vi "lj_obtain_resources.vi"(8 "error in (no error)":errorcluster) -> (0 "error out":errorcluster, 3 "LabJackRes":T1)   [LabVIEW 2025, in "LabJackEKG.lvlib"]
uses:
  LabJackEKG.lvlib
  Typedefs/LabJackGlobalResources.ctl
  Typedefs/CounterQueues.ctl
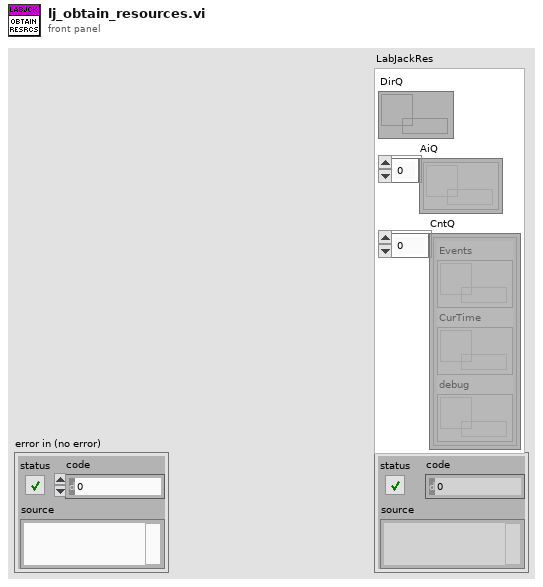
[diagram p1: front panel]
types:
  T1 = typedef "LabJackEKG.lvlib/LabJackGlobalResources.ctl" = cluster{"DirQ":refnum<queue>, "AiQ":refnum<queue>[], "CntQ":T2[]}
  T2 = typedef "LabJackEKG.lvlib/CounterQueues.ctl" = cluster{"Events":refnum<queue>, "CurTime":refnum<queue>, "debug":refnum<queue>}
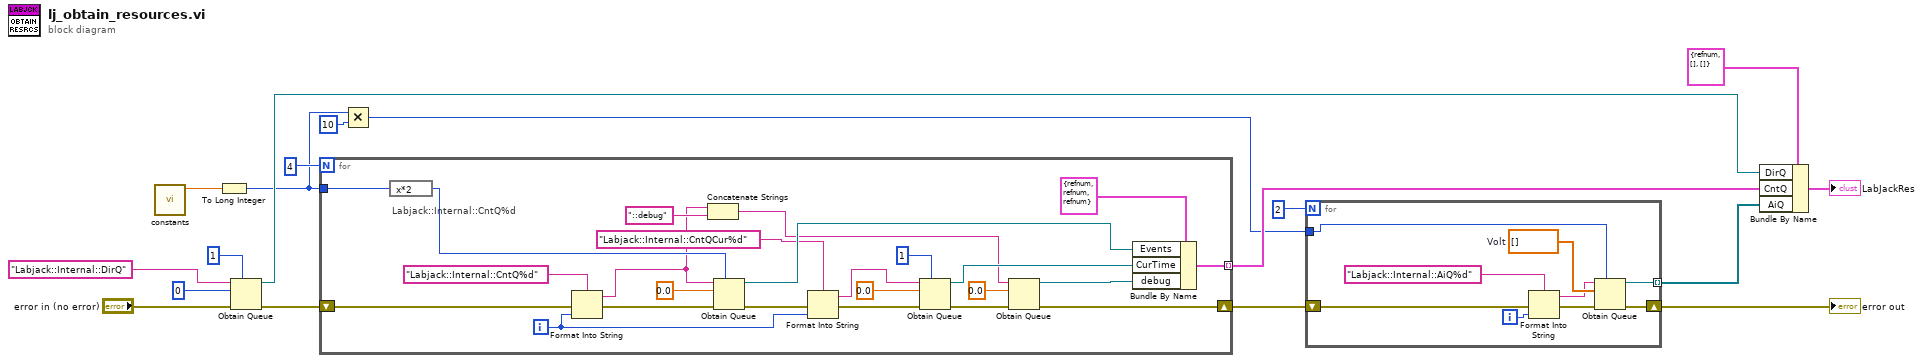
[diagram p0: block diagram]
diagram:
  n1 = call "constants.vi"() -> ("Sampling Frequency [Hz]"=w2:dbl)  [unwired: 10 in, 1 out]
  n2 = To Long Integer(number=w2) -> (32bit integer=w4:i32)
  n3 = Obtain Queue(max queue size (-1, unlimited)=1, name (unnamed)="Labjack::Internal::DirQ", element data type=i64 0, error in (no error)="error in (no error)") -> (queue out=w5:refnum<queue>, error out=w14:errorcluster)  [unwired: 1 in, 1 out]
  n4 = for {
    N: 4 -> [_]
    tunnel: [w35] -> w9 mode=indexing
    shift-right: [w29] -> w13
    shift-left: w14 -> [w40]
    tunnel: w4 -> [w33]
    i -> [w19]
    # "Labjack::Internal::CntQ%d"
    n5 = expression code="x*2"(w33) -> (w32:i32)
    n6 = Format Into String(format string="Labjack::Internal::CntQ%d", error in=w40, w19) -> (resulting string=w23:string, error out=w39:errorcluster)  [unwired: 1 in]
    n7 = Concatenate Strings(w23, "::debug" ("string")) -> (w24:string)
    n8 = Obtain Queue(max queue size (-1, unlimited)=w32, name (unnamed)=w23, element data type=0.0, error in (no error)=w39) -> (queue out=w34:refnum<queue>, error out=w42:errorcluster)  [unwired: 1 in, 1 out]
    n9 = Format Into String(format string="Labjack::Internal::CntQCur%d", error in=w42, w19) -> (resulting string=w20:string, error out=w22:errorcluster)  [unwired: 1 in]
    n10 = Obtain Queue(max queue size (-1, unlimited)=1, name (unnamed)=w20, element data type=0.0, error in (no error)=w22) -> (queue out=w31:refnum<queue>, error out=w30:errorcluster)  [unwired: 1 in, 1 out]
    n11 = Obtain Queue(name (unnamed)=w24, element data type=0.0, error in (no error)=w30) -> (queue out=w28:refnum<queue>, error out=w29:errorcluster)  [unwired: 2 in, 1 out]
    n12 = Bundle By Name(cluster=T2 {"Events"=refnum, "CurTime"=refnum, "debug"=refnum} ("CntQ 2"), "Events"=w34, "CurTime"=w31, "debug"=w28) -> (w35:T2)
  }
  n13 = Multiply(x=w4, y=10 ("max queue size (-1, unlimited)")) -> (x*y=w3:i32)
  n14 = for {
    N: 2 -> [_]
    tunnel: [w50] -> w8 mode=indexing
    shift-right: [w49] -> w12
    shift-left: w13 -> [w48]
    tunnel: w3 -> [w43]
    i -> [w46]
    w51 = dbl[] []  # Volt
    n15 = Format Into String(format string="Labjack::Internal::AiQ%d", error in=w48, w46) -> (resulting string=w44:string, error out=w47:errorcluster)  [unwired: 1 in]
    n16 = Obtain Queue(max queue size (-1, unlimited)=w43, name (unnamed)=w44, element data type=w51, error in (no error)=w47) -> (queue out=w50:refnum<queue>, error out=w49:errorcluster)  [unwired: 1 in, 1 out]
  }
  "error out" <- w12
  n17 = Bundle By Name(cluster=T1 {"DirQ"=refnum, "AiQ"=[], "CntQ"=[]} ("LabJackRes"), "DirQ"=w5, "CntQ"=w9, "AiQ"=w8) -> (→"LabJackRes":T1)
